vi "load class.vi"(8 "error in":errorcluster, 9 "available class paths":path[](array[path]), 10 "available class names":string[](array[string]), 11 "Class Name":string) -> (0 "error out":errorcluster, 3 "Object Out":refnum<class>)   [LabVIEW 2013, in "class discovery singleton.lvlib"]
uses:
  plugin discovery singleton/class discovery singleton.lvlib
  <vilib>/NI/Tag Bus Module Framework/root configuration/TBM configuration.lvclass
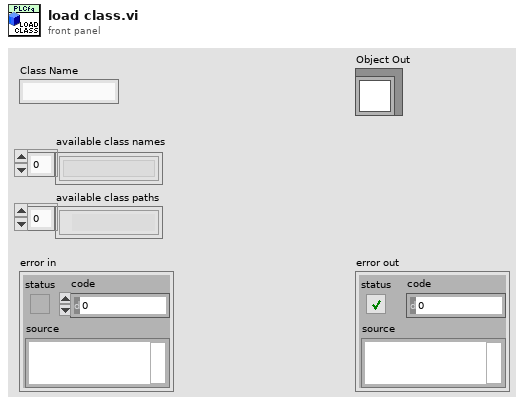
[diagram p1: front panel]
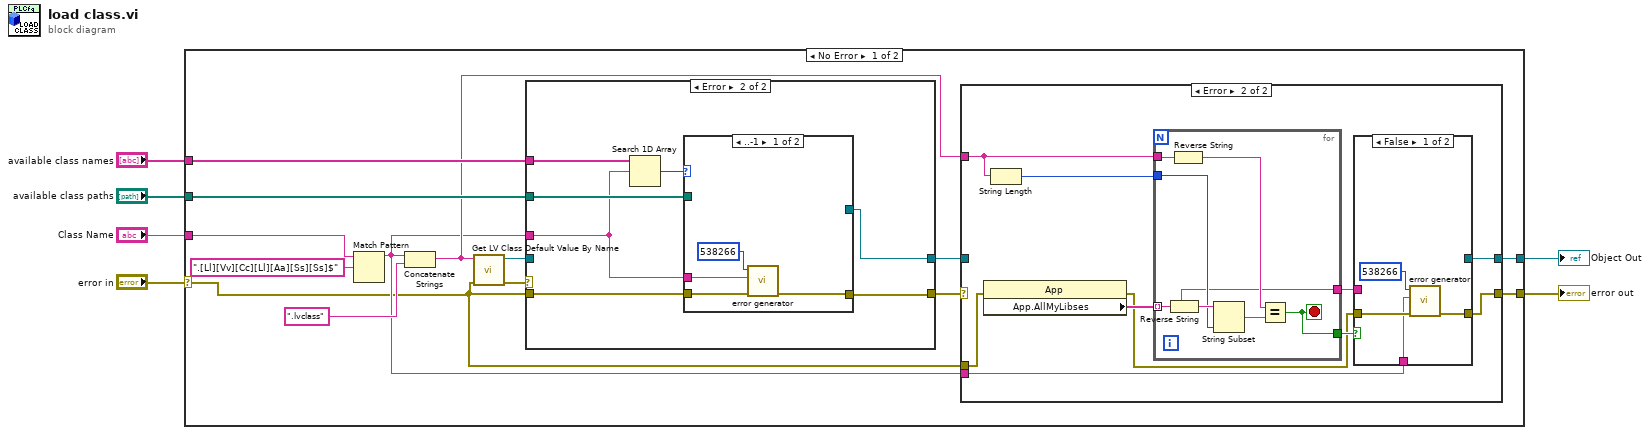
[diagram p0: block diagram]
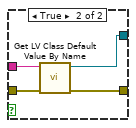
[diagram p3: hidden frame]
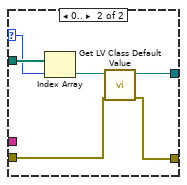
[diagram p5: hidden frame]
diagram:
  n1 = case shown="No Error" "error in" {
    selector: "error in" -> [w7 w67]
    tunnel: "Class Name" -> [w16 _]
    tunnel: [w13 _] -> w3
    tunnel: [w11 w67] -> w4
    tunnel: "available class paths" -> [w18 _]
    tunnel: "available class names" -> [w17 _]
    frame No Error {
      n2 = Match Pattern(string=w16, regular expression=".[Ll][Vv][Cc][Ll][Aa][Ss][Ss]$") -> (before substring=w8:string)  [unwired: 1 in, 3 out]
      n3 = Concatenate Strings(w8, ".lvclass" ("string")) -> (w9:string)
      n4 = call <vilib>:"Get LV Class Default Value By Name.vi"("error in (no error)"=w7, "class name"=w9) -> ("error out"=w20:errorcluster, "object"=w19:refnum<class>)  [unwired: 8 in]
      n5 = case shown="Error" w20 {
        selector: w20 -> [w49 _]
        tunnel: w19 -> [w48 _]
        tunnel: w8 -> [_ w50]
        tunnel: [w49 w55] -> w10
        tunnel: [w48 w56] -> w12
        tunnel: w18 -> [_ w52]
        tunnel: w17 -> [_ w54]
        tunnel: w7 -> [_ w51]
        frame No Error {
        }
        frame Error {
          n6 = Search 1D Array(1D array=w54, element=w50) -> (index of element=w53:i32)  [unwired: 1 in]
          n7 = case shown="..-1" w53 {
            selector: w53 -> [_ w62]
            tunnel: [w59 w66] -> w55
            tunnel: [_ w65] -> w56
            tunnel: w52 -> [_ w64]
            tunnel: w51 -> [w60 w61]
            tunnel: w50 -> [w57 _]
            frame ..-1 {
              n8 = call <vilib>:"error generator.vi"("error in"=w60, "append error message"=w57, "error code (0)"=538266) -> ("error out"=w59:errorcluster)  [unwired: 8 in]
            }
            frame 0.. {
              n9 = Index Array(array=w64, index=w62) -> (element=w63:path)
              n10 = call <vilib>:"Get LV Class Default Value.vi"("error in (no error)"=w61, "class path"=w63) -> ("error out"=w66:errorcluster, "object"=w65:refnum<class>)  [unwired: 8 in]
            }
          }
        }
      }
      n11 = case shown="Error" w10 {
        selector: w10 -> [w21 _]
        tunnel: [w22 w24] -> w13
        tunnel: w12 -> [w22 _]
        tunnel: [w21 w25] -> w11
        tunnel: w7 -> [_ w32]
        tunnel: w9 -> [_ w30]
        tunnel: w8 -> [_ w23]
        frame No Error {
        }
        frame Error {
          n12 = property class="App"(error in=w32) -> (error out=w26:errorcluster, "App.AllMyLibses"=w31:string[])  [unwired: 1 in, 1 out]
          n13 = String Length(string=w30) -> (length=w29:i32)
          n14 = for {
            tunnel: w31 -> [w42] mode=indexing
            tunnel: w30 -> [w47]
            tunnel: w29 -> [w45]
            tunnel: [w42] -> w28
            tunnel: [w41] -> w27
            stop <- w41 stop-if-true
            n15 = Reverse String(1:w42) -> (0:w46:string)
            n16 = Reverse String(1:w47) -> (0:w43:string)
            n17 = String Subset(string=w46, length (rest)=w45) -> (substring=w44:string)  [unwired: 1 in]
            n18 = Equal?(x=w43, y=w44) -> (x = y?=w41:bool)
          }
          n19 = case shown="False" w27 {
            tunnel: w28 -> [_ w40]
            tunnel: w26 -> [w34 w39]
            tunnel: [w35 w38] -> w25
            tunnel: [_ w37] -> w24
            tunnel: w23 -> [w33 _]
            frame False {
              n20 = call <vilib>:"error generator.vi"("error in"=w34, "append error message"=w33, "error code (0)"=538266) -> ("error out"=w35:errorcluster)  [unwired: 8 in]
            }
            frame True {
              n21 = call <vilib>:"Get LV Class Default Value By Name.vi"("error in (no error)"=w39, "class name"=w40) -> ("error out"=w38:errorcluster, "object"=w37:refnum<class>)  [unwired: 8 in]
            }
          }
        }
      }
    }
    frame Error {
    }
  }
  "error out" <- w4
  "Object Out" <- w3
